vi "Bindata&descr to img.vi"(8 "error in (no error)":errorcluster, 9 "bindata_descr index":i32, 11 "Bindata & descr in":T2) -> (0 "error out":errorcluster, 3 "img out":T1)   [LabVIEW 2018, in "LabView-0mq-Jl_Roundtrip_lib.lvlib"]
uses:
  LabView-0mq-Jl_Roundtrip_lib.lvlib
  Bindata&description.ctl
  Bindata description.ctl
  <vilib>/picture/picture.llb/imagedata.ctl
  <vilib>/Utility/error.llb/Error Cluster From Error Code.vi
  <vilib>/ErrorRing/Error Ring.xnode
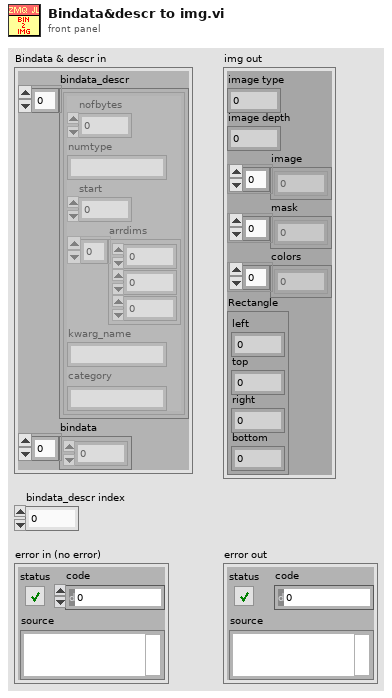
[diagram p1: front panel]
types:
  T1 = typedef "imagedata.ctl" = cluster{"image type":i32, "image depth":i32, "image":u8[], "mask":u8[], "colors":u32[], "Rectangle":cluster{"left":i16, "top":i16, "right":i16, "bottom":i16}}
  T2 = typedef "Bindata&description.ctl" = cluster{"bindata_descr":T3[], "bindata":u8[]}
  T3 = typedef "LabView-0mq-Jl_Roundtrip_lib.lvlib/Bindata description.ctl" = cluster{"nofbytes":i32, "numtype":string, "start":i32, "arrdims":i32[], "kwarg_name":string, "category":string}
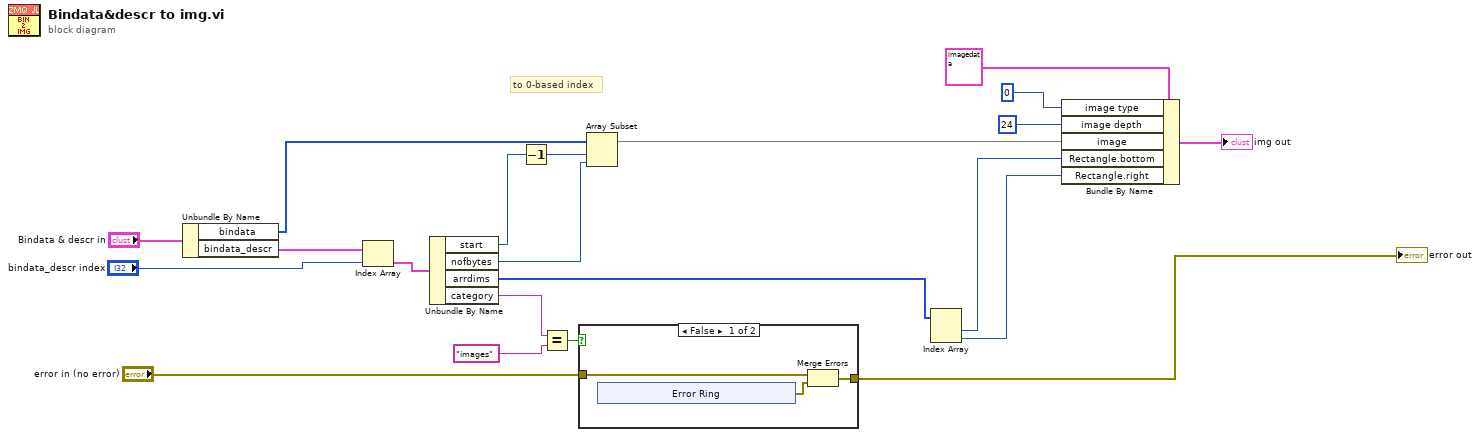
[diagram p0: block diagram]
diagram:
  # "to 0-based index"
  n1 = Unbundle By Name("Bindata & descr in") -> ("bindata"=w18:u8[], "bindata_descr"=w15:T3[])
  n2 = Index Array(array=w15, index="bindata_descr index") -> (element=w17:T3)
  n3 = Unbundle By Name(w17) -> ("start"=w3:i32, "nofbytes"=w2:i32, "arrdims"=w19:i32[], "category"=w7:string)
  n4 = Decrement(x=w3) -> (x-1=w1:i32)
  n5 = Equal?(x=w7, y="images") -> (x = y?=w8:bool)
  n6 = case shown="False" w8 {
    tunnel: [w23 w30] -> w5
    tunnel: "error in (no error)" -> [w24 w30]
    frame False {
      n7 = xnode "Error Ring"() -> ("error out"=w22:errorcluster)
      n8 = Merge Errors(w24, w22) -> (w23:errorcluster)
    }
    frame True {
    }
  }
  "error out" <- w5
  n9 = Array Subset(array=w18, index=w1, length=w2) -> (w4:u8[])
  n10 = Index Array(array=w19) -> (element #1=w20:i32, element #2=w21:i32)  [unwired: 2 in]
  n11 = Bundle By Name(cluster=T1 {"image type"=0, "image depth"=24, "image"=array[196608 elements], "mask"=[], "colors"=[], "Rectangle"={"left"=0, "top"=0, "right"=256, "bottom"=256}} ("img in"), "image type"=i16 0, "image depth"=24, "image"=w4, "Rectangle.bottom"=w20, "Rectangle.right"=w21) -> (→"img out":T1)
